vi "FilterHemisphere.vi"(9 "Queue timeout (ms)":i32=200, 10 "NotifierReff":T2, 11 "Hemisphere Queue Cluster":T1) -> ()   [LabVIEW 2013]
doc: "Performs and filtering that we want (default is no filtering) and writes the data to the notifier. If no data is in the queue this VI times out after 'Queue timeout (ms)' has passed and nothing is written to the notifier.\n\nEric Schneider, March 2014"
uses:
  Data/TypeDefs/Notifiers.ctl
  Data/TypeDefs/UTM Location.ctl
  Data/TypeDefs/Sail Set Suggestions.ctl
  Data/TypeDefs/Rudder Set Suggestions.ctl
  Data/TypeDefs/OverrideInformation.ctl
  Data/TypeDefs/OverrideMode.ctl
  Data/TypeDefs/MotorSetup.ctl
  Data/TypeDefs/DynamixelSetupInfo.ctl
  Data/TypeDefs/AirmarStatus.ctl
  Data/TypeDefs/HardwareOnline.ctl
  Data/TypeDefs/DynamixelCycleTracker.ctl
  Data/TypeDefs/RC Input Values.ctl
  Classes/Missions/GenericMission/GenericMission.lvclass
  Classes/Waypoint/Waypoint.lvclass
  Data/TypeDefs/GPS-Compass Queue Cluster.ctl
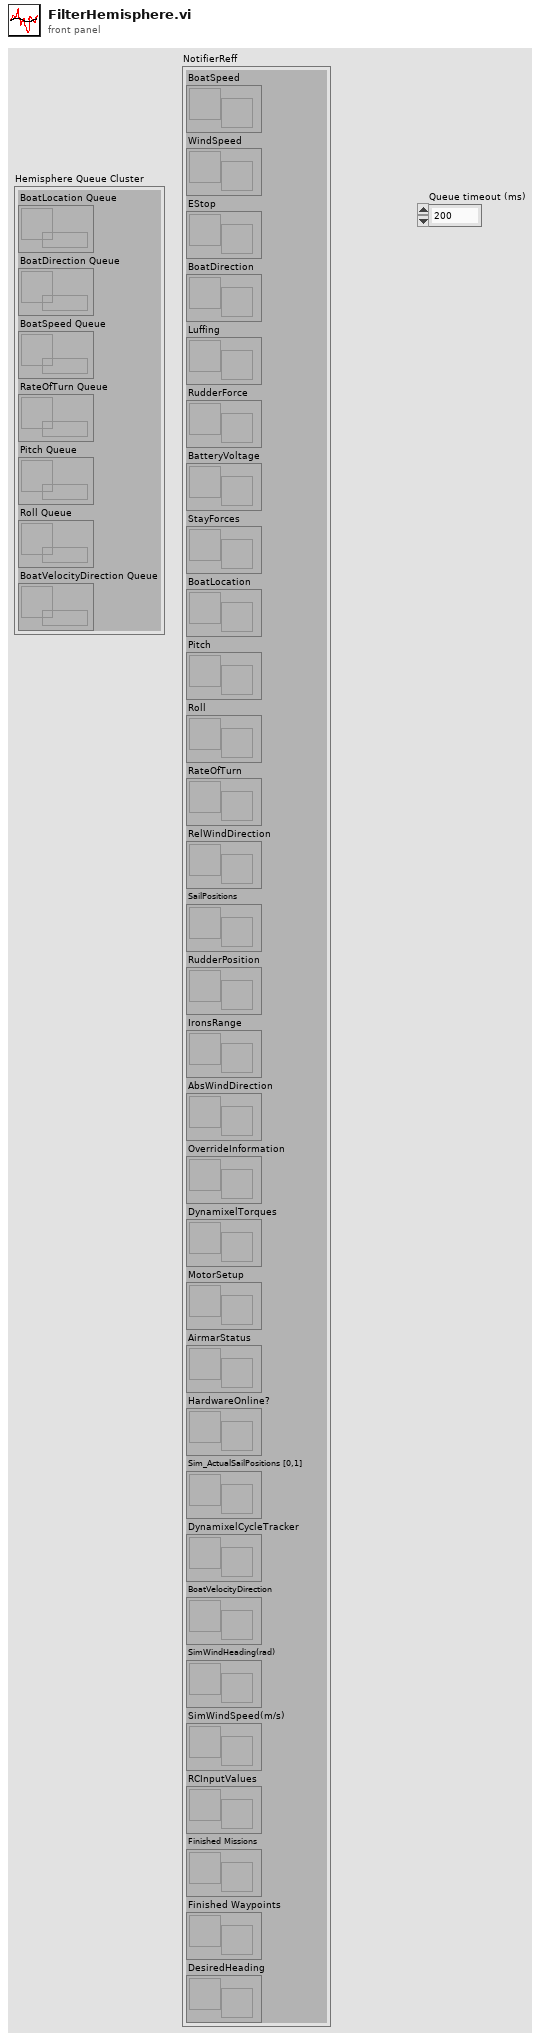
[diagram p1: front panel]
types:
  T1 = typedef "GPS-Compass Queue Cluster.ctl" = cluster{"BoatLocation Queue":refnum<queue>, "BoatDirection Queue":refnum<queue>, "BoatSpeed Queue":refnum<queue>, "RateOfTurn Queue":refnum<queue>, "Pitch Queue":refnum<queue>, "Roll Queue":refnum<queue>, "BoatVelocityDirection Queue ":refnum<queue>}
  T2 = typedef "Notifiers.ctl" = cluster{"BoatSpeed":refnum<notifier>, "WindSpeed":refnum<notifier>, "EStop":refnum<notifier>, "BoatDirection":refnum<notifier>, "Luffing":refnum<notifier>, "RudderForce":refnum<notifier>, "BatteryVoltage":refnum<notifier>, "StayForces":refnum<notifier>, "BoatLocation":refnum<notifier>, "Pitch":refnum<notifier>, "Roll":refnum<notifier>, "RateOfTurn":refnum<notifier>, "RelWindDirection":refnum<notifier>, "SailPositions":refnum<notifier>, "RudderPosition":refnum<notifier>, "IronsRange":refnum<notifier>, "AbsWindDirection":refnum<notifier>, "OverrideInformation":refnum<notifier>, "DynamixelTorques":refnum<notifier>, "MotorSetup":refnum<notifier>, "AirmarStatus":refnum<notifier>, "HardwareOnline?":refnum<notifier>, "Sim_ActualSailPositions [0,1]":refnum<notifier>, "DynamixelCycleTracker":refnum<notifier>, "BoatVelocityDirection":refnum<notifier>, "SimWindHeading(rad)":refnum<notifier>, "SimWindSpeed(m/s)":refnum<notifier>, "RCInputValues":refnum<notifier>, "Finished Missions":refnum<notifier>, "Finished Waypoints":refnum<notifier>, "DesiredHeading":refnum<notifier>}
  T3 = typedef "UTM Location.ctl" = cluster{"UTM Zone":dbl, "Hemisphere":enum16{"North", "South"}, "East":dbl, "North":dbl}
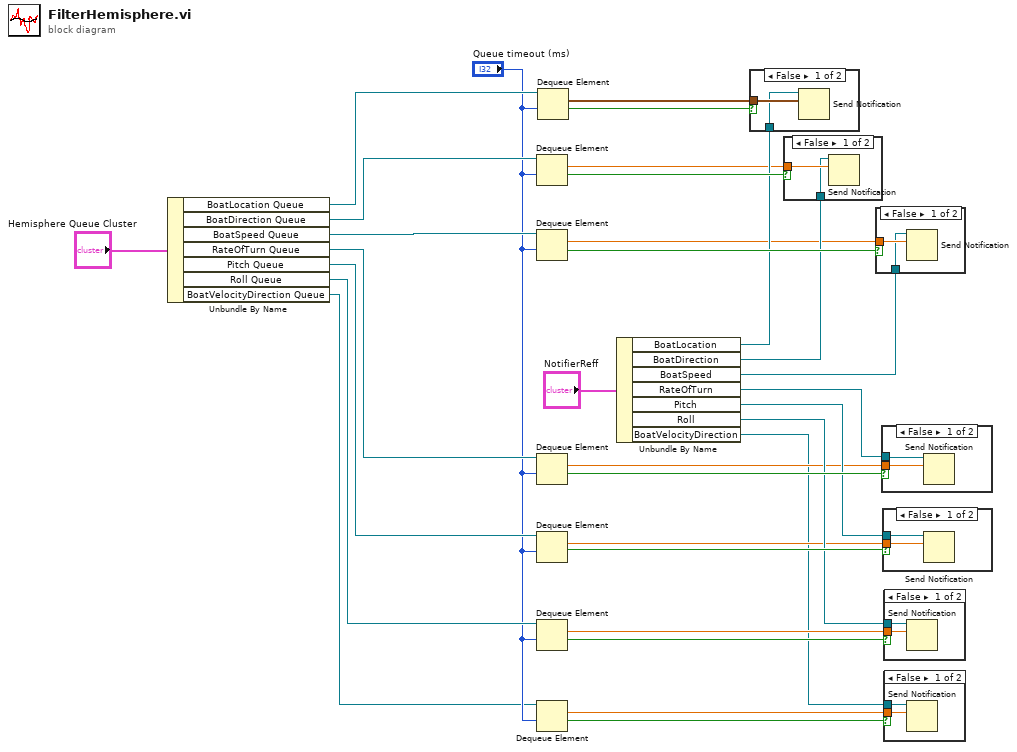
[diagram p0: block diagram]
diagram:
  n1 = Unbundle By Name("Hemisphere Queue Cluster") -> ("BoatLocation Queue"=w7:refnum<queue>, "BoatDirection Queue"=w8:refnum<queue>, "BoatSpeed Queue"=w9:refnum<queue>, "RateOfTurn Queue"=w10:refnum<queue>, "Pitch Queue"=w11:refnum<queue>, "Roll Queue"=w12:refnum<queue>, "BoatVelocityDirection Queue"=w4:refnum<queue>)
  n2 = Dequeue Element(queue=w8, timeout in ms (-1)="Queue timeout (ms)") -> (element=w14:dbl, timed out?=w27:bool)  [unwired: 1 in, 2 out]
  n3 = Dequeue Element(queue=w9, timeout in ms (-1)="Queue timeout (ms)") -> (element=w16:dbl, timed out?=w28:bool)  [unwired: 1 in, 2 out]
  n4 = Dequeue Element(queue=w10, timeout in ms (-1)="Queue timeout (ms)") -> (element=w15:dbl, timed out?=w29:bool)  [unwired: 1 in, 2 out]
  n5 = Dequeue Element(queue=w11, timeout in ms (-1)="Queue timeout (ms)") -> (element=w17:dbl, timed out?=w30:bool)  [unwired: 1 in, 2 out]
  n6 = Dequeue Element(queue=w12, timeout in ms (-1)="Queue timeout (ms)") -> (element=w18:dbl, timed out?=w31:bool)  [unwired: 1 in, 2 out]
  n7 = Dequeue Element(queue=w4, timeout in ms (-1)="Queue timeout (ms)") -> (element=w2:dbl, timed out?=w3:bool)  [unwired: 1 in, 2 out]
  n8 = Dequeue Element(queue=w7, timeout in ms (-1)="Queue timeout (ms)") -> (element=w13:T3, timed out?=w26:bool)  [unwired: 1 in, 2 out]
  n9 = Unbundle By Name("NotifierReff") -> ("BoatLocation"=w20:refnum<notifier>, "BoatDirection"=w21:refnum<notifier>, "BoatSpeed"=w22:refnum<notifier>, "RateOfTurn"=w23:refnum<notifier>, "Pitch"=w24:refnum<notifier>, "Roll"=w25:refnum<notifier>, "BoatVelocityDirection"=w1:refnum<notifier>)
  n10 = case shown="False" w26 {
    tunnel: w13 -> [w33 _]
    tunnel: w20 -> [w32 _]
    frame False {
      n11 = Send Notification(notification=w33, notifier=w32) -> ()  [unwired: 1 in, 2 out]
    }
    frame True {
    }
  }
  n12 = case shown="False" w27 {
    tunnel: w14 -> [w35 _]
    tunnel: w21 -> [w34 _]
    frame False {
      n13 = Send Notification(notification=w35, notifier=w34) -> ()  [unwired: 1 in, 2 out]
    }
    frame True {
    }
  }
  n14 = case shown="False" w28 {
    tunnel: w16 -> [w37 _]
    tunnel: w22 -> [w36 _]
    frame False {
      n15 = Send Notification(notification=w37, notifier=w36) -> ()  [unwired: 1 in, 2 out]
    }
    frame True {
    }
  }
  n16 = case shown="False" w29 {
    tunnel: w15 -> [w39 _]
    tunnel: w23 -> [w38 _]
    frame False {
      n17 = Send Notification(notification=w39, notifier=w38) -> ()  [unwired: 1 in, 2 out]
    }
    frame True {
    }
  }
  n18 = case shown="False" w30 {
    tunnel: w17 -> [w41 _]
    tunnel: w24 -> [w40 _]
    frame False {
      n19 = Send Notification(notification=w41, notifier=w40) -> ()  [unwired: 1 in, 2 out]
    }
    frame True {
    }
  }
  n20 = case shown="False" w31 {
    tunnel: w18 -> [w43 _]
    tunnel: w25 -> [w42 _]
    frame False {
      n21 = Send Notification(notification=w43, notifier=w42) -> ()  [unwired: 1 in, 2 out]
    }
    frame True {
    }
  }
  n22 = case shown="False" w3 {
    tunnel: w2 -> [w45 _]
    tunnel: w1 -> [w44 _]
    frame False {
      n23 = Send Notification(notification=w45, notifier=w44) -> ()  [unwired: 1 in, 2 out]
    }
    frame True {
    }
  }
